vi "server.Add Response (Custom Error).vi"(4 "message":string, 5 "id value":string, 6 "code":i32, 7 "jsonrpc":string="2.0", 8 "error in (no error)":errorcluster, 10 "data":refnum<class "JSON Null.lvclass">, 11 "Server in":refnum<class "JSONRPC Server.lvclass">) -> (0 "error out":errorcluster, 1 "response string":string, 3 "Server out":refnum<class "JSONRPC Server.lvclass">)   [LabVIEW 2016, in "JSONRPC Server.lvclass"]
uses:
  JSONRPC Server.lvclass
  <vilib>/NI/JSON Support for LabVIEW/JSON Data Classes/JSON Datatype/JSON Null.lvclass
  error/error.lvclass
  error/error.Write code.vi
  error/error.Write message.vi
  error/error.Write data.vi
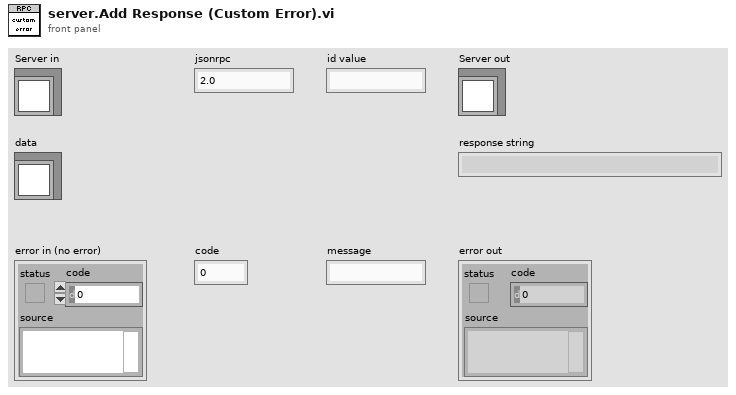
[diagram p1: front panel]
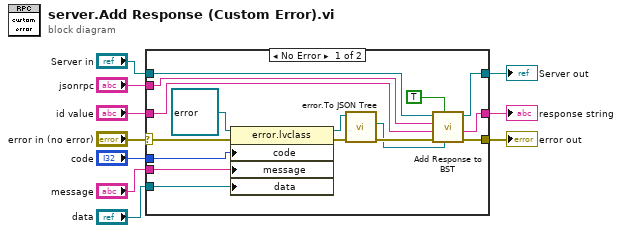
[diagram p0: block diagram]
diagram:
  n1 = case shown="No Error" "error in (no error)" {
    selector: "error in (no error)" -> [w22 w28]
    tunnel: [w18 w28] -> w9
    tunnel: [w25 w27] -> w7
    tunnel: "Server in" -> [w26 w27]
    tunnel: "code" -> [w17 _]
    tunnel: "message" -> [w16 _]
    tunnel: "data" -> [w11 _]
    tunnel: "jsonrpc" -> [w14 _]
    tunnel: "id value" -> [w13 _]
    tunnel: [w12 _] -> w1
    frame No Error {
      n2 = property class="error.lvclass"(reference=refnum<class "error.lvclass"> refnum ("error.lvclass"), error in=w22, "code"=w17, "message"=w16, "data"=w11) -> (reference out=w21:refnum<class "error.lvclass">, error out=w20:errorcluster)
      n3 = call "error.To JSON Tree.vi"("error in (no error)"=w20, "error in"=w21) -> ("error out"=w19:errorcluster, "JSON out"=w15:refnum<class "JSON Null.lvclass">)  [unwired: 7 in, 1 out]
      n4 = call "Add Response to BST.vi"("JSON in"=w15, "error"=TRUE, "error in (no error)"=w19, "id value"=w13, "jsonrpc"=w14, "Server in"=w26) -> ("error out"=w18:errorcluster, "response string"=w12:string, "Server out"=w25:refnum<class "JSONRPC Server.lvclass">)  [unwired: 2 in, 1 out]
    }
    frame Error {
    }
  }
  "error out" <- w9
  "Server out" <- w7
  "response string" <- w1
